vi "Actor Core.vi"(8 "error in":errorcluster, 11 "Configuration Window in":refnum<class "Configuration Window.lvclass">) -> (0 "error out":errorcluster, 3 "Actor out":refnum<class "Actor.lvclass">)   [LabVIEW 2018, in "Configuration Window.lvlib" / "Configuration Window.lvclass"]
doc: "The user interface for this panel.\n\n----\nPlease see the following web address for additional documentation and tutorial information:\nhttp://www.mooregoodideas.com/mgi-panel-manager/\n\nAuthor: Derek Trepanier\n\nCopyright (c) 2018, Moore Good Ideas, Inc.\n\nAll rights reserved.\n\nRedistribution and use in source and binary forms, with or without modification, are permitted provided that the following conditions are met:\n\n * Redistributions of source code must retain the above copyright notice, this list of conditions and the following disclaimer.\n * Redistributions in binary form must reproduce the above copyright notice, this list of conditions and the following disclaimer in the documentation and/or other materials provided with the distribution.\n * Neither the name of Moore Good Ideas, Inc. nor the names of its contributors may be used to endorse or promote products derived from this software without specific prior written permission.\n\nTHIS SOFTWARE IS PROVIDED BY THE COPYRIGHT HOLDERS AND CONTRIBUTORS \"AS IS\" AND ANY EXPRESS OR IMPLIED WARRANTIES, INCLUDING, BUT NOT LIMITED TO, THE IMPLIED WARRANTIES OF MERCHANTABILITY AND FITNESS FOR A PARTICULAR PURPOSE ARE DISCLAIMED. IN NO EVENT SHALL THE COPYRIGHT OWNER OR CONTRIBUTORS BE LIABLE FOR ANY DIRECT, INDIRECT, INCIDENTAL, SPECIAL, EXEMPLARY, OR CONSEQUENTIAL DAMAGES (INCLUDING, BUT NOT LIMITED TO, PROCUREMENT OF SUBSTITUTE GOODS OR SERVICES; LOSS OF USE, DATA, OR PROFITS; OR BUSINESS INTERRUPTION) HOWEVER CAUSED AND ON ANY THEORY OF LIABILITY, WHETHER IN CONTRACT, STRICT LIABILITY, OR TORT (INCLUDING NEGLIGENCE OR OTHERWISE) ARISING IN ANY WAY OUT OF THE USE OF THIS SOFTWARE, EVEN IF ADVISED OF THE POSSIBILITY OF SUCH DAMAGE."
uses:
  Configuration Window.lvclass
  C:/Program Files (x86)/National Instruments/LabVIEW 2018/vi.lib/MGI/Panel Manager/Panel Actor/Panel Actor/Panel Actor.lvclass
  <vilib>/ActorFramework/Actor/Actor.lvclass
  Configuration Window.lvclass/Configuration Window.ctl
  Framework/Framework/Framework.lvclass
  <vilib>/MGI/Panel Manager/Panel Actor/Panel Actor/Panel Actor.lvclass
panel:
  in  "Cancel":bool
  in  "Save":bool
  in  "Tab Control":enum32{"Main", "Image"}(tab)
  in  "mp3 Folder Path":path
  in  "Language":u16(ring)
  in  "_res_pngs Folder Path":path
  in  "_res_data Folder Path":path
  in  "Reset to Steam Path":bool
  out "c Name":string="<c> Point:"
  out "o Name":string="<o> Point:"
  out "i Name":string="<i> Box:"
  out "b Name":string="<b> Box:"
  out "w Name":string="<w> Point:"
  out "bp Name":string="<bp> Point:"
  in  "c Size":i32 caption="Size"
  in  "c Enable":bool caption="Enable"
  in  "c Color":u32(colorbox) caption="Color"
  in  "o Size":i32 caption="Size"
  in  "o Enable":bool caption="Enable"
  in  "o Color":u32(colorbox) caption="Color"
  in  "i Fill Color":u32(colorbox) caption="Fill Color"
  in  "i Enable":bool caption="Enable"
  in  "i Border Color":u32(colorbox) caption="Border Color"
  in  "b Fill Color":u32(colorbox) caption="Fill Color"
  in  "b Enable":bool caption="Enable"
  in  "b Border Color":u32(colorbox) caption="Border Color"
  in  "w Enable":bool caption="Enable"
  in  "w Color":u32(colorbox) caption="Color"
  in  "w Size":i32 caption="Size"
  in  "bp Enable":bool caption="Enable"
  in  "bp Color":u32(colorbox) caption="Color"
  in  "bp Size":i32 caption="Size"
  in  "CP Enable":bool caption="Enable"
  in  "CP Color":u32(colorbox) caption="Color"
  in  "CP Size":i32 caption="Size"
  out "CP Name":string="Center Point:"
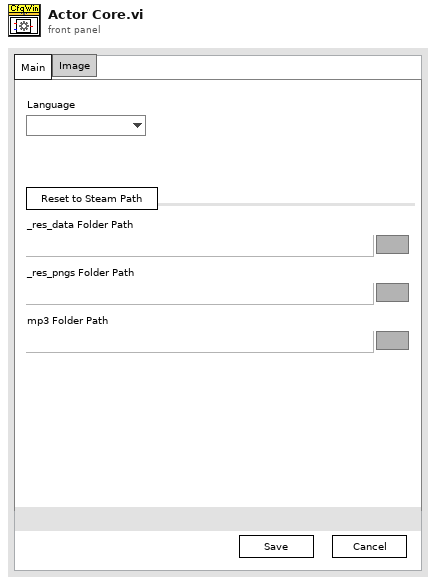
[diagram p1: front panel]
types:
  T1 = cluster{"Reset to Steam Path":refnum<vi>, "_res_data Folder Path":refnum<vi>, "_res_pngs Folder Path":refnum<vi>, "mp3 Folder Path":refnum<vi>}
  T2 = cluster{"CP Name":refnum<vi>, "CP Size":refnum<vi>, "CP Color":refnum<vi>, "CP Enable":refnum<vi>}
  T3 = cluster{"bp Name":refnum<vi>, "bp Size":refnum<vi>, "bp Color":refnum<vi>, "bp Enable":refnum<vi>}
  T4 = cluster{"w Name":refnum<vi>, "w Size":refnum<vi>, "w Color":refnum<vi>, "w Enable":refnum<vi>}
  T5 = cluster{"b Name":refnum<vi>, "b Fill Color":refnum<vi>, "b Border Color":refnum<vi>, "b Enable":refnum<vi>}
  T6 = cluster{"i Name":refnum<vi>, "i Fill Color":refnum<vi>, "i Border Color":refnum<vi>, "i Enable":refnum<vi>}
  T7 = cluster{"o Name":refnum<vi>, "o Size":refnum<vi>, "o Color":refnum<vi>, "o Enable":refnum<vi>}
  T8 = cluster{"c Name":refnum<vi>, "c Size":refnum<vi>, "c Color":refnum<vi>, "c Enable":refnum<vi>}
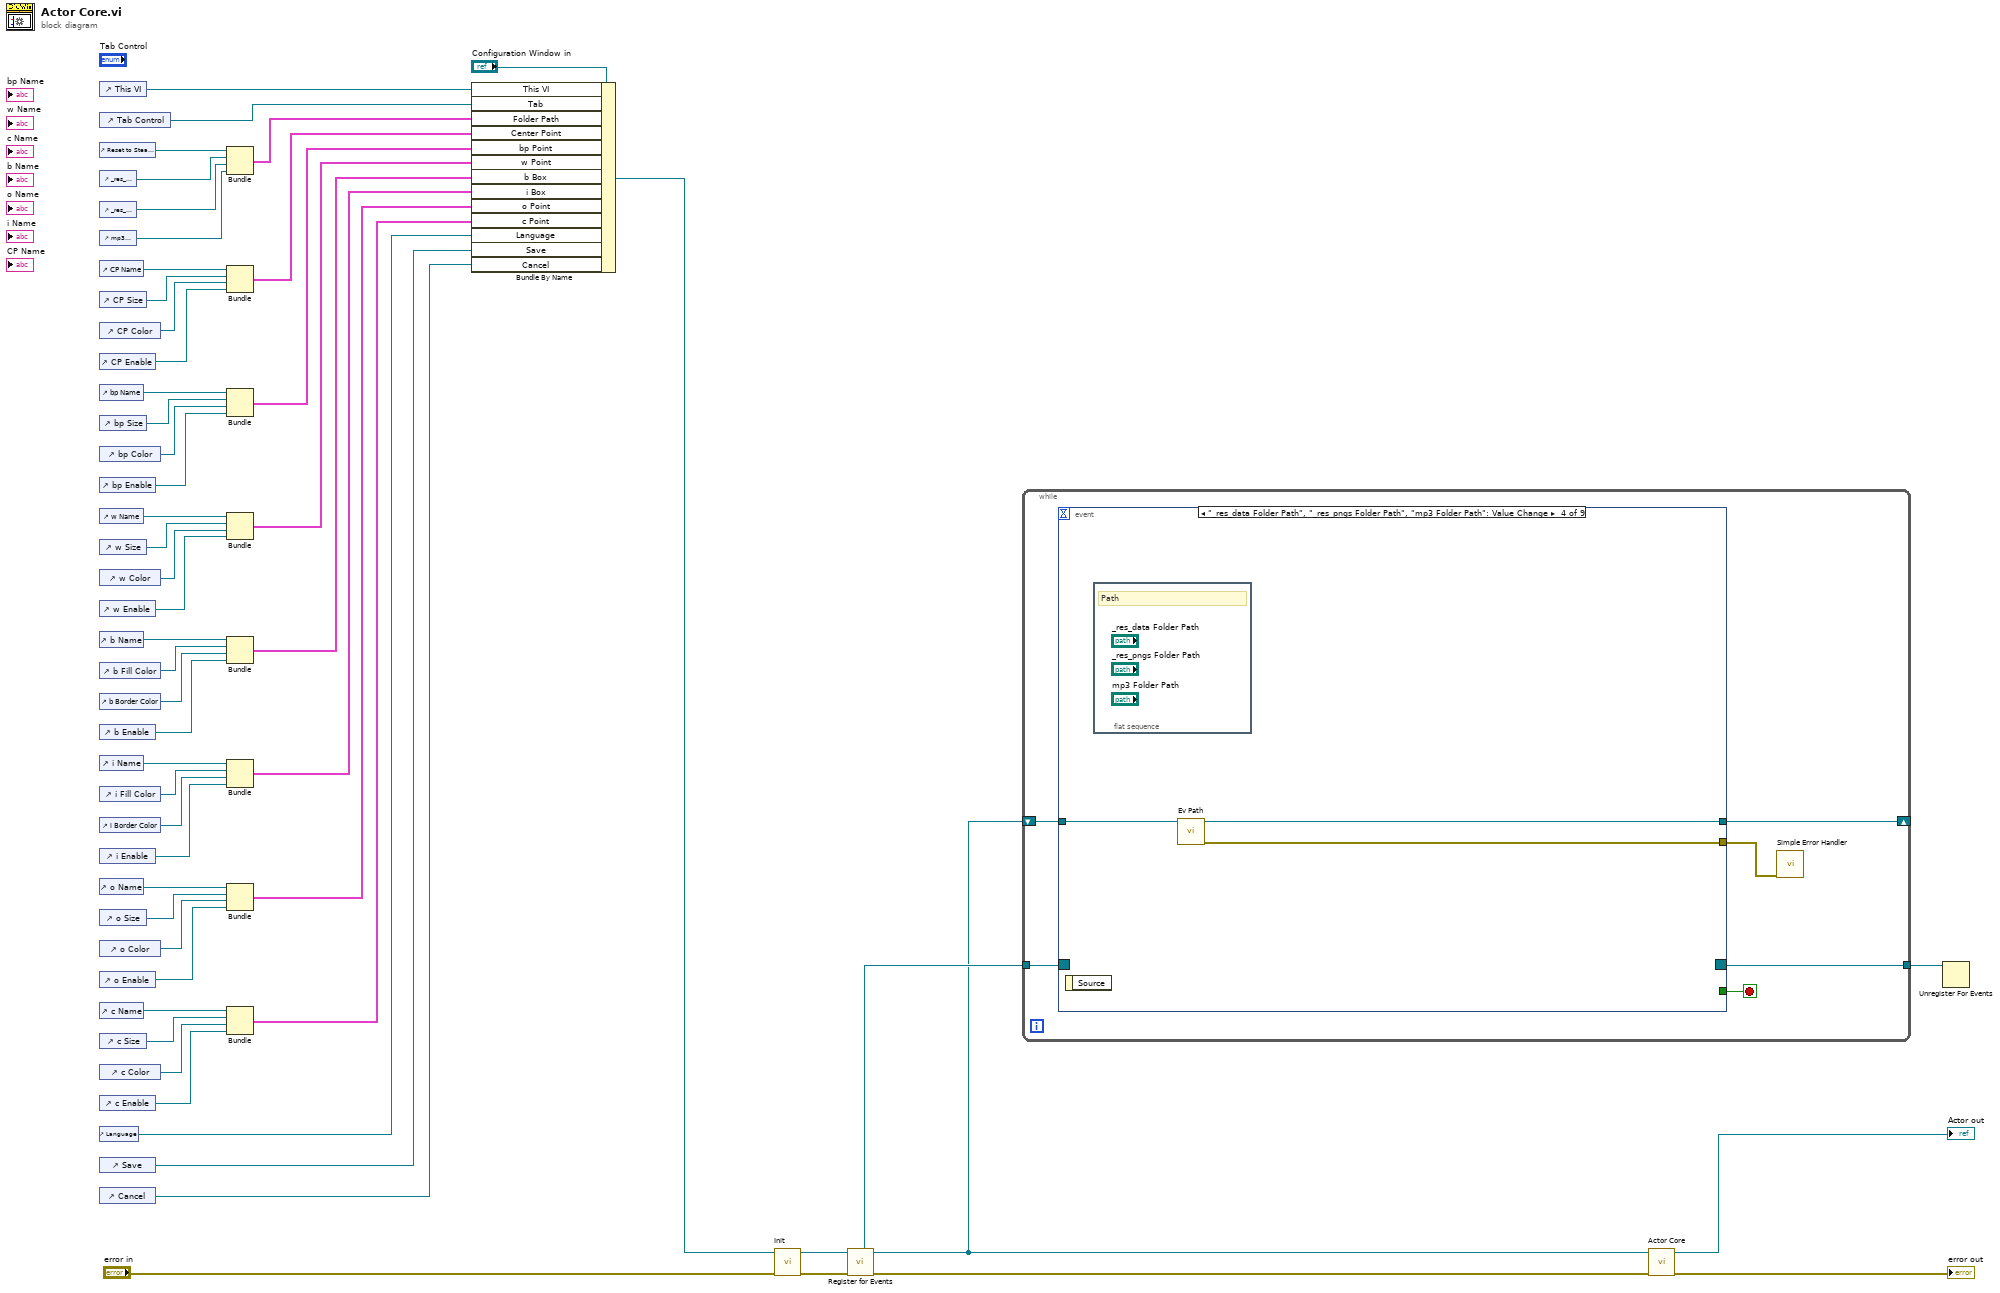
[diagram p0: block diagram]
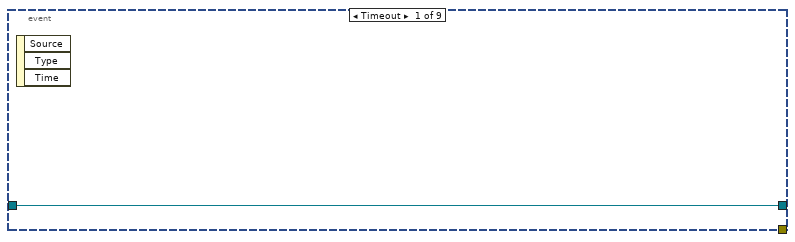
[diagram p2: hidden frame]
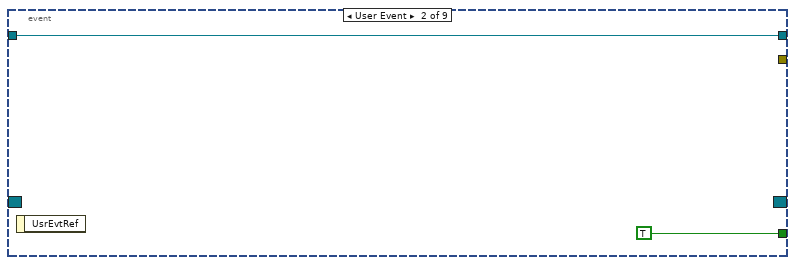
[diagram p3: hidden frame]
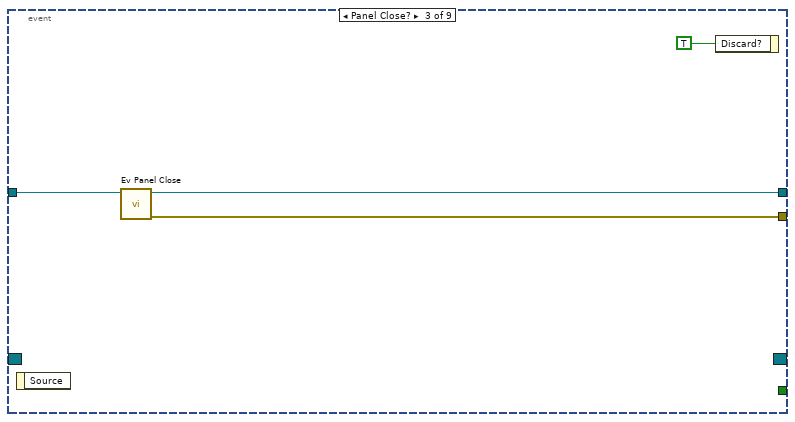
[diagram p4: hidden frame]
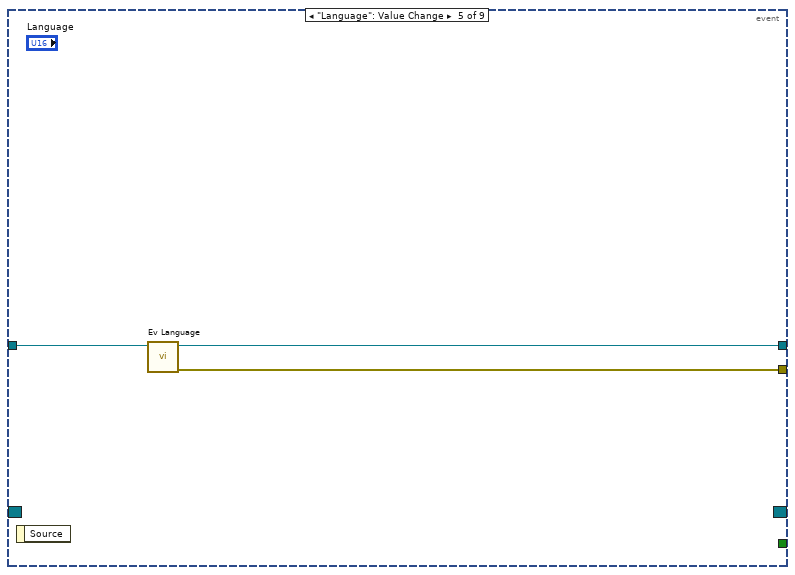
[diagram p5: hidden frame]
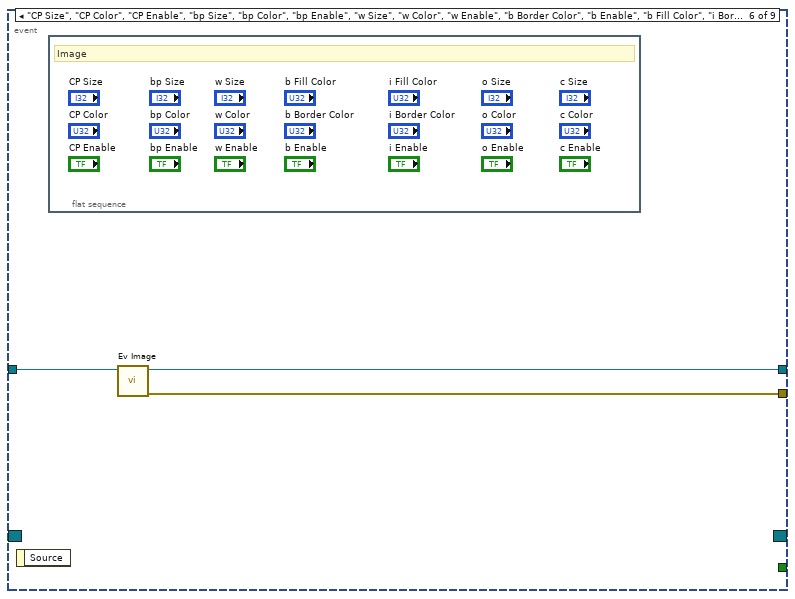
[diagram p6: hidden frame]
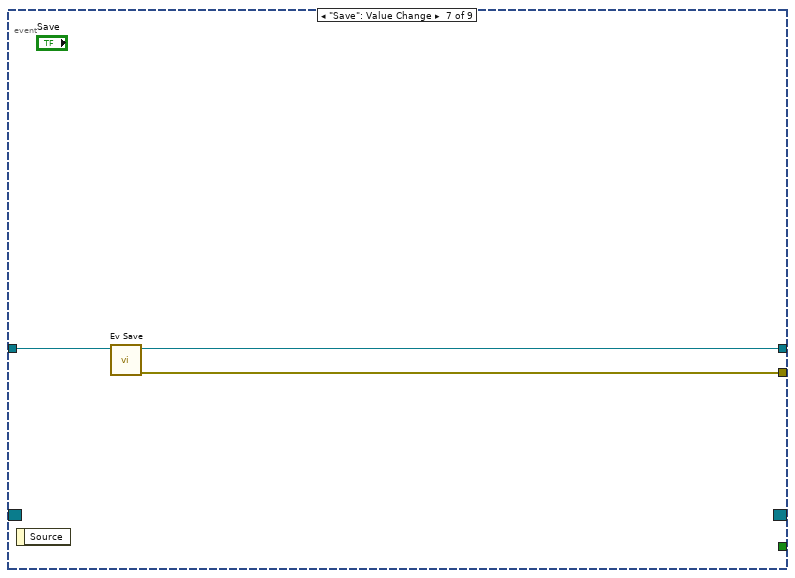
[diagram p7: hidden frame]
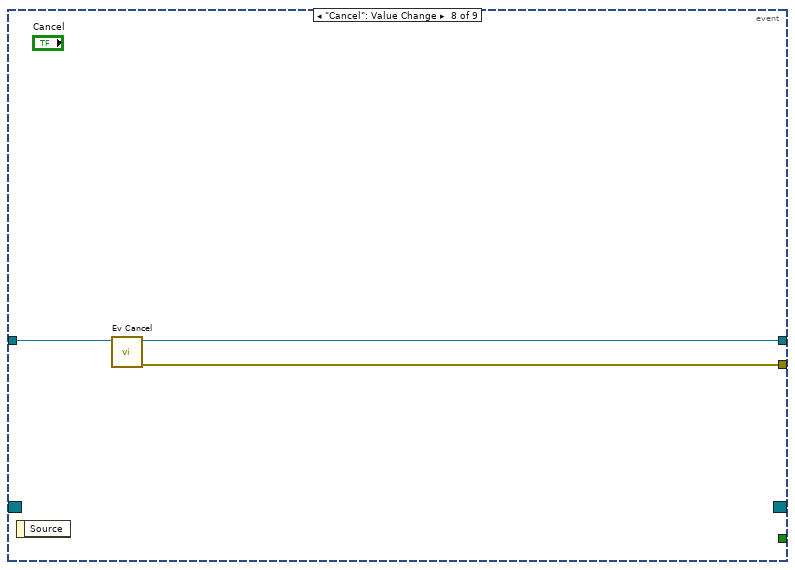
[diagram p8: hidden frame]
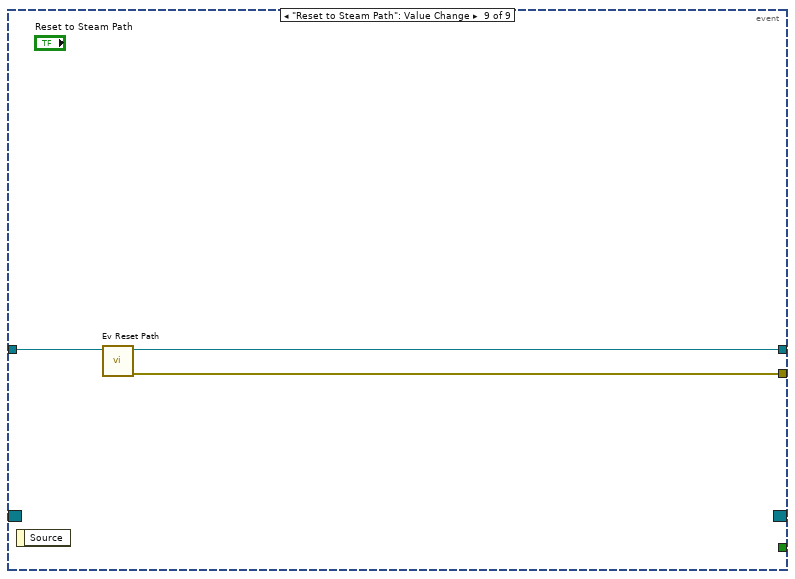
[diagram p9: hidden frame]
diagram:
  n1 = control-ref of="This VI"() -> (w49:refnum<vi>)
  n2 = control-ref of="Tab Control"() -> (w5:refnum<vi>)
  n3 = control-ref of="Reset to Steam Path"() -> (w2:refnum<vi>)
  n4 = control-ref of="_res_data Folder Path"() -> (w48:refnum<vi>)
  n5 = control-ref of="_res_pngs Folder Path"() -> (w47:refnum<vi>)
  n6 = control-ref of="mp3 Folder Path"() -> (w1:refnum<vi>)
  n7 = control-ref of="CP Name"() -> (w6:refnum<vi>)
  n8 = control-ref of="CP Size"() -> (w45:refnum<vi>)
  n9 = control-ref of="CP Color"() -> (w44:refnum<vi>)
  n10 = control-ref of="CP Enable"() -> (w43:refnum<vi>)
  n11 = control-ref of="bp Name"() -> (w7:refnum<vi>)
  n12 = control-ref of="bp Size"() -> (w41:refnum<vi>)
  n13 = control-ref of="bp Color"() -> (w40:refnum<vi>)
  n14 = control-ref of="bp Enable"() -> (w39:refnum<vi>)
  n15 = control-ref of="w Name"() -> (w8:refnum<vi>)
  n16 = control-ref of="w Size"() -> (w37:refnum<vi>)
  n17 = control-ref of="w Color"() -> (w36:refnum<vi>)
  n18 = control-ref of="w Enable"() -> (w35:refnum<vi>)
  n19 = control-ref of="b Name"() -> (w9:refnum<vi>)
  n20 = control-ref of="b Fill Color"() -> (w33:refnum<vi>)
  n21 = control-ref of="b Border Color"() -> (w32:refnum<vi>)
  n22 = control-ref of="b Enable"() -> (w31:refnum<vi>)
  n23 = control-ref of="i Name"() -> (w10:refnum<vi>)
  n24 = control-ref of="i Fill Color"() -> (w29:refnum<vi>)
  n25 = control-ref of="i Border Color"() -> (w28:refnum<vi>)
  n26 = control-ref of="i Enable"() -> (w27:refnum<vi>)
  n27 = control-ref of="o Name"() -> (w11:refnum<vi>)
  n28 = control-ref of="o Size"() -> (w25:refnum<vi>)
  n29 = control-ref of="o Color"() -> (w24:refnum<vi>)
  n30 = control-ref of="o Enable"() -> (w23:refnum<vi>)
  n31 = control-ref of="c Name"() -> (w12:refnum<vi>)
  n32 = control-ref of="c Size"() -> (w21:refnum<vi>)
  n33 = control-ref of="c Color"() -> (w20:refnum<vi>)
  n34 = control-ref of="c Enable"() -> (w19:refnum<vi>)
  n35 = control-ref of="Language"() -> (w13:refnum<vi>)
  n36 = control-ref of="Save"() -> (w4:refnum<vi>)
  n37 = control-ref of="Cancel"() -> (w3:refnum<vi>)
  n38 = Bundle("Reset to Steam Path"=w2, "_res_data Folder Path"=w48, "_res_pngs Folder Path"=w47, "mp3 Folder Path"=w1) -> (w46:T1)  [unwired: 1 in]
  n39 = Bundle("CP Name"=w6, "CP Size"=w45, "CP Color"=w44, "CP Enable"=w43) -> (w42:T2)  [unwired: 1 in]
  n40 = Bundle("bp Name"=w7, "bp Size"=w41, "bp Color"=w40, "bp Enable"=w39) -> (w38:T3)  [unwired: 1 in]
  n41 = Bundle("w Name"=w8, "w Size"=w37, "w Color"=w36, "w Enable"=w35) -> (w34:T4)  [unwired: 1 in]
  n42 = Bundle("b Name"=w9, "b Fill Color"=w33, "b Border Color"=w32, "b Enable"=w31) -> (w30:T5)  [unwired: 1 in]
  n43 = Bundle("i Name"=w10, "i Fill Color"=w29, "i Border Color"=w28, "i Enable"=w27) -> (w26:T6)  [unwired: 1 in]
  n44 = Bundle("o Name"=w11, "o Size"=w25, "o Color"=w24, "o Enable"=w23) -> (w22:T7)  [unwired: 1 in]
  n45 = Bundle("c Name"=w12, "c Size"=w21, "c Color"=w20, "c Enable"=w19) -> (w18:T8)  [unwired: 1 in]
  n46 = Bundle By Name(cluster="Configuration Window in", "This VI"=w49, "Tab"=w5, "Folder Path"=w46, "Center Point"=w42, "bp Point"=w38, "w Point"=w34, "b Box"=w30, "i Box"=w26, "o Point"=w22, "c Point"=w18, "Language"=w13, "Save"=w4, "Cancel"=w3) -> (w17:refnum<class "Configuration Window.lvclass">)
  n47 = call "Init.vi"("error in (no error)"="error in", "Configuration Window in"=w17) -> ("error out"=w15:errorcluster, "Configuration Window out"=w16:refnum<class "Configuration Window.lvclass">)  [unwired: 8 in]
  n48 = call <vilib>:"Register for Events.vi"("Error In"=w15, "Panel Actor in"=w16) -> ("Error Out"=w53:errorcluster, "Panel Actor out"=w51:refnum<class "Configuration Window.lvclass">, "Pnl Actor"=w52:refnum<event-registration>)  [unwired: 6 in, 1 out]
  n49 = while {
    tunnel: [w61] -> w54
    tunnel: w52 -> [w60]
    shift-right: [w58] -> _
    shift-left: w51 -> [w59]
    stop <- w62 stop-if-true
    n50 = event shown="[3] \"_res_data Folder Path\", \"_res_pngs Folder Path\", \"mp3 Folder Path\": Value Change" {
      selector: w60 -> [_ _ _ _ _ _ _ _ _]
      dyn-events: [_ _ _ _ _ _ _ _ _] -> w61
      timeout: _ -> [_ _ _ _ _ _ _ _ _]
      tunnel: [_ TRUE _ _ _ _ _ _ _] -> w62
      tunnel: w59 -> [w63 w64 w68 w72 w75 w78 w81 w84 w87]
      tunnel: [w63 w64 w66 w70 w73 w77 w79 w82 w85] -> w58
      tunnel: [_ _ w67 w71 w74 w76 w80 w83 w86] -> w57
      event Timeout {
        n51 = event-data() -> ()  [unwired: 1 in, 3 out]
      }
      event User Event {
        n52 = event-data() -> ()  [unwired: 1 in, 1 out]
      }
      event Panel Close? {
        n53 = event-data() -> ()  [unwired: 1 in, 1 out]
        n54 = call "Ev Panel Close.vi"("Configuration Window in"=w68) -> ("error out"=w67:errorcluster, "Configuration Window out"=w66:refnum<class "Configuration Window.lvclass">)  [unwired: 9 in]
        n55 = event-data("Discard?"=TRUE) -> ()  [unwired: 1 in, 1 out]
      }
      event "_res_data Folder Path", "_res_pngs Folder Path", "mp3 Folder Path": Value Change {
        n56 = event-data() -> ()  [unwired: 1 in, 1 out]
        n57 = flat-sequence {
          frame #0 {
            # "Path"
          }
        }
        n58 = call "Ev Path.vi"("Configuration Window in"=w72) -> ("error out"=w71:errorcluster, "Configuration Window out"=w70:refnum<class "Configuration Window.lvclass">)  [unwired: 9 in]
      }
      event "Language": Value Change {
        n59 = event-data() -> ()  [unwired: 1 in, 1 out]
        n60 = call "Ev Language.vi"("Configuration Window in"=w75) -> ("error out"=w74:errorcluster, "Configuration Window out"=w73:refnum<class "Configuration Window.lvclass">)  [unwired: 9 in]
      }
      event "CP Size", "CP Color", "CP Enable", "bp Size", "bp Color", "bp Enable", "w Size", "w Color", "w Enable", "b Border Color", "b Enable", "b Fill Color", "i Border Color", "i Enable", "i Fill Color", "o Color", "o Enable", "o Size", "c Color", "c Enable", "c Size": Value Change {
        n61 = event-data() -> ()  [unwired: 1 in, 1 out]
        n62 = flat-sequence {
          frame #0 {
            # "Image"
          }
        }
        n63 = call "Ev Image.vi"("Configuration Window in"=w78) -> ("error out"=w76:errorcluster, "Configuration Window out"=w77:refnum<class "Configuration Window.lvclass">)  [unwired: 9 in]
      }
      event "Save": Value Change {
        n64 = event-data() -> ()  [unwired: 1 in, 1 out]
        n65 = call "Ev Save.vi"("Configuration Window in"=w81) -> ("error out"=w80:errorcluster, "Configuration Window out"=w79:refnum<class "Configuration Window.lvclass">)  [unwired: 9 in]
      }
      event "Cancel": Value Change {
        n66 = event-data() -> ()  [unwired: 1 in, 1 out]
        n67 = call "Ev Cancel.vi"("Configuration Window in"=w84) -> ("error out"=w83:errorcluster, "Configuration Window out"=w82:refnum<class "Configuration Window.lvclass">)  [unwired: 9 in]
      }
      event "Reset to Steam Path": Value Change {
        n68 = event-data() -> ()  [unwired: 1 in, 1 out]
        n69 = call "Ev Reset Path.vi"("Configuration Window in"=w87) -> ("error out"=w86:errorcluster, "Configuration Window out"=w85:refnum<class "Configuration Window.lvclass">)  [unwired: 9 in]
      }
    }
    n70 = call <vilib>:"Simple Error Handler.vi"("error in (no error)"=w57) -> ()  [unwired: 4 in, 5 out]
  }
  n71 = call-parent "Actor Core.vi"("error in"=w53, "Panel Actor in"=w51) -> ("error out"=→"error out":errorcluster, "Actor out"=→"Actor out":refnum<class "Actor.lvclass">)  [unwired: 8 in]
  n72 = Unregister For Events(event registration refnum=w54) -> ()  [unwired: 1 in, 1 out]
